vi "Launcher Preparation.vi"(2 "Elevation":dbl, 3 "Shooting Motors":dbl) -> ()   [LabVIEW 2012]
uses:
  BotStatus.vi
  Motors Values.vi
  <vilib>/express/express arith-compare/Formula/XNode/ExpressFormulaBlockNode.xnode
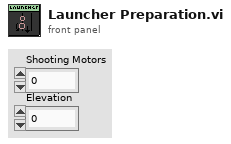
[diagram p1: front panel]
types:
  T1 = cluster{"Middle":bool, "InCannon":bool, "InFlipper":bool, "FlipperAtPlace":bool, "Bottom":bool, "FrisbeeDirection":bool}
  T2 = typedef "WPI_EncoderDevRef.ctl" = cluster{"DevStatus":errorcluster, "EncoderIndex":T3, "CounterIndex":T4, "DistancePerCount":dbl, "Decoding Type":T5}
  T3 = typedef "FPGA_EncoderIdx.ctl" = enum8{"Enc 0", "Enc 1", "Enc 2", "Enc 3", "Invalid"}
  T4 = typedef "FPGA_CounterCtrSystemIndex.ctl" = enum8{"Ctr 0", "Ctr 1", "Ctr 2", "Ctr 3", "Ctr 4", "Ctr 5", "Ctr 6", "Ctr 7", "Invalid"}
  T5 = typedef "WPI_EncoderType.ctl" = enum16{"1x", "2x", "4x"}
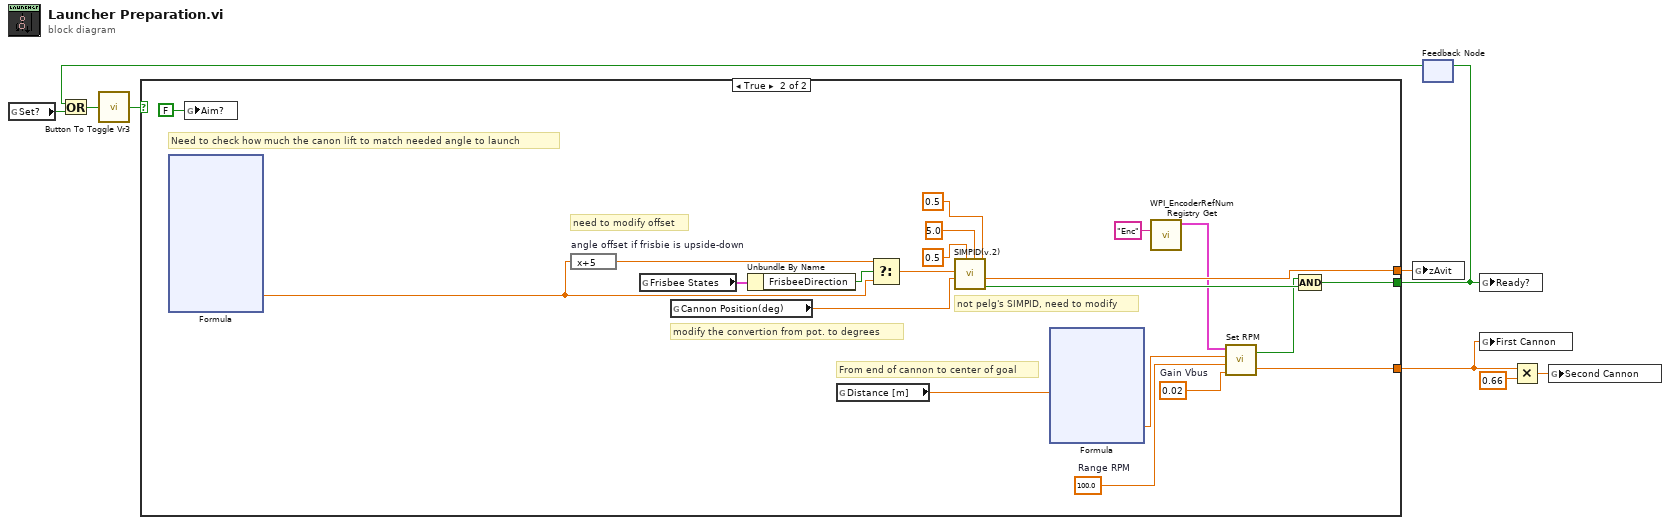
[diagram p0: block diagram]
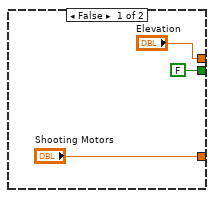
[diagram p2: hidden frame]
diagram:
  n1 = global read "BotStatus.vi" "Set?"() -> (w2:bool)
  n2 = feedback #1() -> (w1:bool)  [unwired: 1 in]
  n3 = Or(x=w1, y=w2) -> (x .or. y?=w5:bool)
  n4 = call "Button To Toggle Vr3.vi"("InValue"=w5) -> ("Result"=w4:bool)
  n5 = case shown="True" w4 {
    tunnel: ["Elevation" w22] -> w7
    tunnel: ["Shooting Motors" w20] -> w6
    tunnel: [FALSE w16] -> w3
    frame False {
    }
    frame True {
      w17 = 0.02  # Gain Vbus
      w18 = 100.0  # Range RPM
      # "From end of cannon to center of goal"
      # "need to modify offset"
      # "not pelg's SIMPID, need to modify"
      # "modify the convertion from pot. to degrees"
      # "Need to check how much the canon lift to match needed angle to launch"
      n6 = xnode "Formula"() -> ("Result"=w28:dbl)  [unwired: 5 in, 1 out]
      n7 = global write "BotStatus.vi" "Aim?"(FALSE ("Centerizing on Target")) -> ()
      n8 = expression code="x+5" "angle offset if frisbie is upside-down"(w28) -> (w27:dbl)
      n9 = global read "BotStatus.vi" "Frisbee States"() -> (w24:T1)
      n10 = global read "BotStatus.vi" "Cannon Position(deg)"() -> (w26:dbl)
      n11 = Unbundle By Name(w24) -> ("FrisbeeDirection"=w23:bool)
      n12 = global read "BotStatus.vi" "Distance [m]"() -> (w25:dbl)
      n13 = Select(t=w27, s=w23, f=w28) -> (s? t:f=w29:dbl)
      n14 = call "SIMPID(v.2).vi"("Range"=0.5, "upper limit"=5.0, "lower limit"=0.5, "Current Point"=w26, "Set Point"=w29) -> ("On Target"=w33:bool, "result"=w22:dbl)  [unwired: 5 in]
      n15 = xnode "Formula"("D"=w25) -> ("Result"=w21:dbl)  [unwired: 2 in, 1 out]
      n16 = call <vilib>:"WPI_EncoderRefNum Registry Get.vi"("refnum name"="Enc") -> ("EncoderDevRef"=w14:T2)  [unwired: 9 in, 1 out]
      n17 = call "Set RPM.vi"("Gain Vbus"=w17, "Range RPM"=w18, "Set Point RPM"=w21, "EncoderDevRef"=w14) -> ("Vbus Out"=w20:dbl, "READY!"=w19:bool)
      n18 = Compound Arithmetic op=AND(w19, w33) -> (w16:bool)
    }
  }
  n19 = global write "Motors Values.vi" "zAvit"(w7) -> ()
  n20 = feedback-in #1(w3) -> ()
  n21 = global write "BotStatus.vi" "Ready?"(w3) -> ()
  n22 = global write "Motors Values.vi" "First Cannon"(w6) -> ()
  n23 = Multiply(x=w6, y=0.66) -> (x*y=w8:dbl)
  n24 = global write "Motors Values.vi" "Second Cannon"(w8) -> ()
